vi "Array Magnitude.vi"(0 "x":dbl[](array[numeric]) format="%.2f", 2 "Mode":u16(ring) items=["Absolute", "Relative"], 5 "y":dbl[](array[numeric]) format="%.2f", 7 "x 2":dbl[](array[numeric]) format="%.2f", 9 "y 2":dbl[](array[numeric]) format="%.2f", 11 "error in (no error)":errorcluster) -> (4 "z":dbl[](array[numeric]) format="%.2f", 15 "error out":errorcluster)   [LabVIEW 2017]
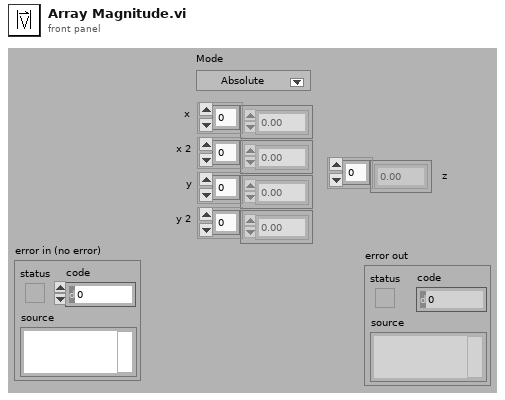
[diagram p1: front panel]
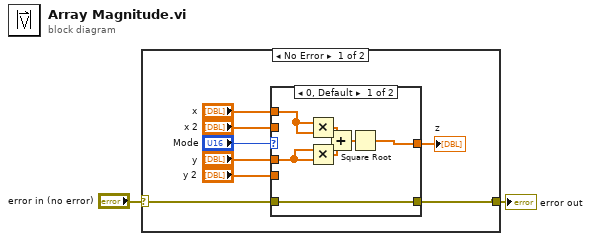
[diagram p0: block diagram]
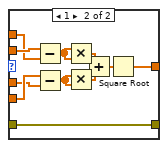
[diagram p2: hidden frame]
diagram:
  n1 = case shown="No Error" "error in (no error)" {
    selector: "error in (no error)" -> [w4 w29]
    tunnel: [w3 w29] -> w1
    frame No Error {
      n2 = case shown="0, Default" "Mode" {
        tunnel: "x" -> [w14 w24]
        tunnel: "y" -> [w13 w20]
        tunnel: [w12 w19] -> w5
        tunnel: "x 2" -> [_ w25]
        tunnel: "y 2" -> [_ w21]
        tunnel: w4 -> [w11 w18]
        tunnel: [w11 w18] -> w3
        frame 0, Default {
          n3 = Multiply(x=w14, y=w14) -> (x*y=w17:dbl[])
          n4 = Multiply(x=w13, y=w13) -> (x*y=w15:dbl[])
          n5 = Add(x=w17, y=w15) -> (x+y=w16:dbl[])
          n6 = Square Root(x=w16) -> (sqrt(x)=w12:dbl[])
        }
        frame 1 {
          n7 = Subtract(x=w25, y=w24) -> (x-y=w23:dbl[])
          n8 = Subtract(x=w21, y=w20) -> (x-y=w22:dbl[])
          n9 = Multiply(x=w23, y=w23) -> (x*y=w28:dbl[])
          n10 = Multiply(x=w22, y=w22) -> (x*y=w26:dbl[])
          n11 = Add(x=w28, y=w26) -> (x+y=w27:dbl[])
          n12 = Square Root(x=w27) -> (sqrt(x)=w19:dbl[])
        }
      }
      "z" <- w5
    }
    frame Error {
    }
  }
  "error out" <- w1
